vi "SW_get_config_of_Zones_and_IO_2.vi"(0 "Sync parameters cluster input":T2={"IO general config."=12, "IO 1 configuration"=1, "IO 2 configuration"=1, "IO 3 configuration"=0, "IO 4 configuration"=0, "Activate ext. RS-232"=0, "IO inversion config."=0, "Sync capability"=0}) -> (1 "Zones out config":u32, 2 "Zones out config bin":bool[](array[boolean]), 3 "Ports IO config (OUT is FALSE)":bool[](array[boolean]), 4 "IO inversion config.":u16)   [LabVIEW 2018, in "Tracker.lvlib"]
uses:
  Tracker.lvlib
  Controls/CTL_IO_params_cluster.ctl
  Controls/CTL_IO_status_indicator.ctl
  <vilib>/Utility/miscctls.llb/LVPointTypeDef.ctl
panel:
  out "IO status indicator":T1
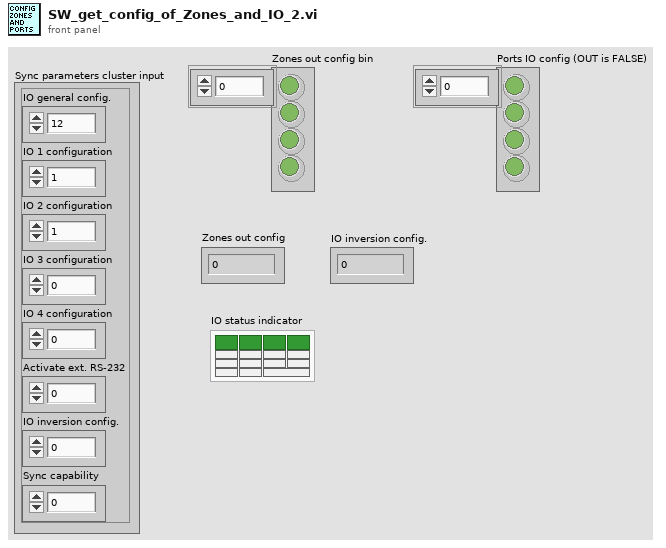
[diagram p1: front panel]
types:
  T1 = typedef "Tracker.lvlib/CTL_IO_status_indicator.ctl" = cluster{"IO1":bool, "IO2":bool, "IO3":bool, "IO4":bool, "St1":bool, "St2":bool, "St3":bool, "St4":bool, "Z1":bool, "Z2":bool, "Z3":bool, "Z4":bool, "Syn1":bool, "Syn2":bool, "RS-232 ext. activated":bool}
  T2 = typedef "Tracker.lvlib/CTL_IO_params_cluster.ctl" = cluster{"IO general config.":u16, "IO 1 configuration":u16, "IO 2 configuration":u16, "IO 3 configuration":u16, "IO 4 configuration":u16, "Activate ext. RS-232":u16, "IO inversion config.":u16, "Sync capability":u8}
  T3 = typedef "LVPointTypeDef.ctl" = cluster{"Horizontal":i16, "Vertical":i16}
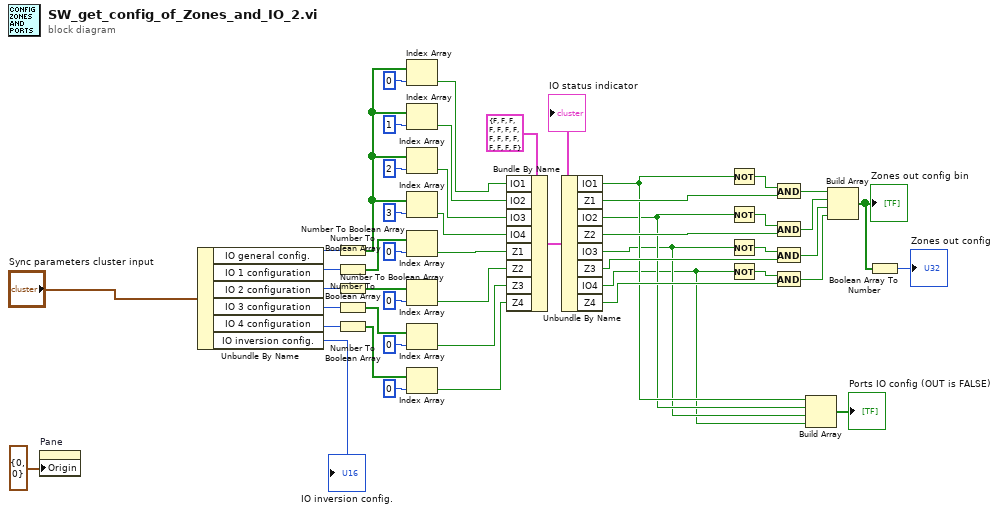
[diagram p0: block diagram]
diagram:
  n1 = property on="Pane" class="Pane"("Origin"=T3 {"Horizontal"=0, "Vertical"=0}) -> ()  [unwired: 2 in, 2 out]
  n2 = Unbundle By Name("Sync parameters cluster input") -> ("IO general config."=w46:u16, "IO 1 configuration"=w40:u16, "IO 2 configuration"=w35:u16, "IO 3 configuration"=w32:u16, "IO 4 configuration"=w31:u16, "IO inversion config."=→"IO inversion config.":u16)
  n3 = Number To Boolean Array(number=w46) -> (Boolean array=w45:bool[])
  n4 = Number To Boolean Array(number=w40) -> (Boolean array=w39:bool[])
  n5 = Number To Boolean Array(number=w35) -> (Boolean array=w36:bool[])
  n6 = Number To Boolean Array(number=w32) -> (Boolean array=w34:bool[])
  n7 = Number To Boolean Array(number=w31) -> (Boolean array=w33:bool[])
  n8 = Index Array(array=w45, index=0) -> (element=w50:bool)
  n9 = Index Array(array=w45, index=1) -> (element=w49:bool)
  n10 = Index Array(array=w45, index=2) -> (element=w48:bool)
  n11 = Index Array(array=w45, index=3) -> (element=w47:bool)
  n12 = Index Array(array=w39, index=0) -> (element=w26:bool)
  n13 = Index Array(array=w36, index=0) -> (element=w25:bool)
  n14 = Index Array(array=w34, index=0) -> (element=w24:bool)
  n15 = Index Array(array=w33, index=0) -> (element=w23:bool)
  n16 = Bundle By Name(cluster=T1 {"IO1"=FALSE, "IO2"=FALSE, "IO3"=FALSE, "IO4"=FALSE, "St1"=FALSE, "St2"=FALSE, "St3"=FALSE, "St4"=FALSE, "Z1"=FALSE, "Z2"=FALSE, "Z3"=FALSE, "Z4"=FALSE, "Syn1"=FALSE, "Syn2"=FALSE, "RS-232 ext. activated"=FALSE} ("IO status indicator"), "IO1"=w50, "IO2"=w49, "IO3"=w48, "IO4"=w47, "Z1"=w26, "Z2"=w25, "Z3"=w24, "Z4"=w23) -> (w14:T1)
  "IO status indicator" <- w14
  n17 = Unbundle By Name(w14) -> ("IO1"=w6:bool, "Z1"=w11:bool, "IO2"=w5:bool, "Z2"=w10:bool, "IO3"=w4:bool, "Z3"=w9:bool, "IO4"=w3:bool, "Z4"=w8:bool)
  n18 = Not(x=w6) -> (.not. x?=w22:bool)
  n19 = Not(x=w5) -> (.not. x?=w21:bool)
  n20 = Not(x=w4) -> (.not. x?=w20:bool)
  n21 = Not(x=w3) -> (.not. x?=w19:bool)
  n22 = And(x=w22, y=w11) -> (x .and. y?=w18:bool)
  n23 = And(x=w21, y=w10) -> (x .and. y?=w17:bool)
  n24 = And(x=w20, y=w9) -> (x .and. y?=w16:bool)
  n25 = And(x=w19, y=w8) -> (x .and. y?=w15:bool)
  n26 = Build Array(w6, w5, w4, w3) -> (→"Ports IO config (OUT is FALSE)":bool[])
  n27 = Build Array(w18, w17, w16, w15) -> (w13:bool[])
  "Zones out config bin" <- w13
  n28 = Boolean Array To Number(Boolean array=w13) -> (number=→"Zones out config":u32)
